vi "CameraSetParams.vi"(8 "error in (no error)":errorcluster, 10 "settings":T2={"exposure"=0.0, "external"=FALSE, "roi"={"left"=0, "top"=0, "right"=0, "bottom"=0}, "frames"=0, "bin_x"=1, "bin_y"=1}, 11 "NIvision in":refnum<class "IMAQdx.lvclass">) -> (0 "error out":errorcluster, 1 "roi_out":T1, 2 "attributes":variant[](array[variant]), 3 "NIvision out":refnum<class "IMAQdx.lvclass">)   [LabVIEW 2010, in "IMAQdx.lvclass"]
uses:
  IMAQdx.lvclass
  subvis/ExposureSettings.ctl
  subvis/ROI_rect.ctl
  <vilib>/vision/driver/IMAQdx.llb/IMAQdx Acquisition Mode.ctl
  IMAQdx.lvclass/IMAQdx.ctl
  <vilib>/vision/driver/NI_Vision_Acquisition_Software.lvlib
  Program Files (x86)/National Instruments/LabVIEW 2010/resource/objmgr/imaqdx.rc
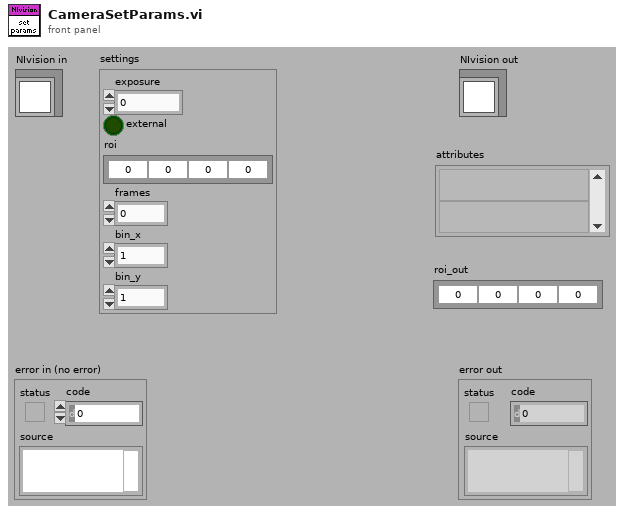
[diagram p1: front panel]
types:
  T1 = typedef "ROI_rect.ctl" = cluster{"left":i32, "top":i32, "right":i32, "bottom":i32}
  T2 = typedef "ExposureSettings.ctl" = cluster{"exposure":dbl, "external":bool, "roi":T1, "frames":i32, "bin_x":u8, "bin_y":u8}
  T3 = typedef "NI_Vision_Acquisition_Software.lvlib/IMAQdx Acquisition Mode.ctl" = enum32{"One Shot", "Continuous"}
  T4 = typedef "IMAQdx.ctl" = refnum<k21>
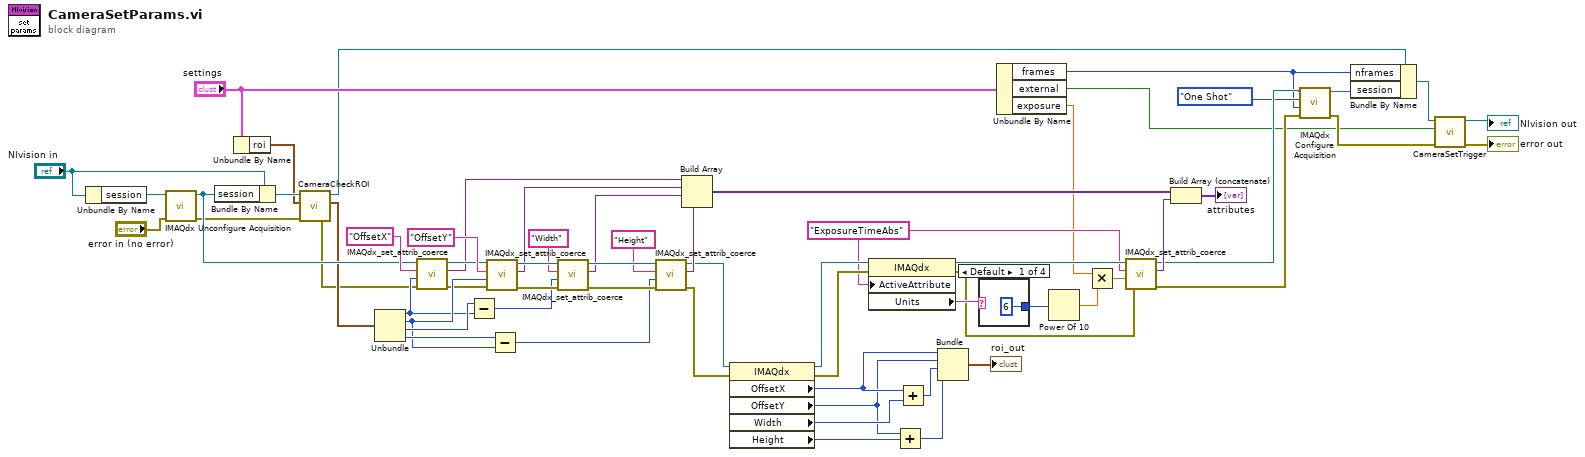
[diagram p0: block diagram]
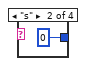
[diagram p2: hidden frame]
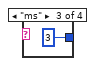
[diagram p3: hidden frame]
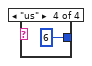
[diagram p4: hidden frame]
diagram:
  w27 = "ExposureTimeAbs" ("ActiveAttribute")
  n1 = Unbundle By Name("NIvision in") -> ("session"=w24:refnum<k21>)
  n2 = call <vilib>:"IMAQdx Unconfigure Acquisition.vi"("error in"="error in (no error)", "Session In"=w24) -> ("error out"=w7:errorcluster, "Session Out"=w13:T4)  [unwired: 8 in]
  n3 = Bundle By Name(cluster="NIvision in", "session"=w13) -> (w11:refnum<class "IMAQdx.lvclass">)
  n4 = Unbundle By Name("settings") -> ("roi"=w9:T1)
  n5 = call-dynamic "CameraCheckROI.vi"("error in (no error)"=w7, "ROI_in"=w9, "IMAQdx in"=w11) -> ("error out"=w6:errorcluster, "ROI_out"=w8:T1, "IMAQdx out"=w10:refnum<class "IMAQdx.lvclass">)  [unwired: 6 in]
  n6 = Unbundle(w8) -> ("left"=w53:i32, "top"=w57:i32, "right"=w63:i32, "bottom"=w60:i32)
  n7 = call "IMAQdx_set_attrib_coerce.vi"("error in"=w6, "value"=w53, "attribute"="OffsetX", "IMAQdx in"=w13) -> ("error out"=w56:errorcluster, "attrib out"=w54:variant, "IMAQdx out"=w55:T4)  [unwired: 1 out]
  n8 = Subtract(x=w63, y=w53) -> (x-y=w48:i32)
  n9 = call "IMAQdx_set_attrib_coerce.vi"("error in"=w56, "value"=w57, "attribute"="OffsetY", "IMAQdx in"=w55) -> ("error out"=w51:errorcluster, "attrib out"=w46:variant, "IMAQdx out"=w52:T4)  [unwired: 1 out]
  n10 = Subtract(x=w60, y=w57) -> (x-y=w47:i32)
  n11 = call "IMAQdx_set_attrib_coerce.vi"("error in"=w51, "value"=w48, "attribute"="Width", "IMAQdx in"=w52) -> ("error out"=w49:errorcluster, "attrib out"=w45:variant, "IMAQdx out"=w50:T4)  [unwired: 1 out]
  n12 = call "IMAQdx_set_attrib_coerce.vi"("error in"=w49, "value"=w47, "attribute"="Height", "IMAQdx in"=w50) -> ("error out"=w32:errorcluster, "attrib out"=w44:variant, "IMAQdx out"=w30:T4)  [unwired: 1 out]
  n13 = Build Array(w54, w46, w45, w44) -> (w41:variant[])
  n14 = property class="IMAQdx"(reference=w30, error in=w32) -> (reference out=w29:T4, error out=w31:errorcluster, "OffsetX"=w38:u32, "OffsetY"=w37:u32, "Width"=w39:u32, "Height"=w40:u32)
  n15 = property class="IMAQdx"(reference=w29, error in=w31, "ActiveAttribute"=w27) -> (reference out=w28:T4, error out=w26:errorcluster, "Units"=w61:string)
  n16 = Add(x=w37, y=w40) -> (x+y=w35:u32)
  n17 = Add(x=w38, y=w39) -> (x+y=w36:u32)
  n18 = Bundle("OffsetX"=w38, "OffsetY"=w37, w36, w35) -> (→"roi_out":cluster{"OffsetX":u32, "OffsetY":u32, u32, u32})  [unwired: 1 in]
  n19 = case shown="Default" w61 {
    tunnel: [6 ("y") 0 ("y") 3 ("y") 6 ("y")] -> w4
    frame Default {
    }
    frame "s" {
    }
    frame "ms" {
    }
    frame "us" {
    }
  }
  n20 = Unbundle By Name("settings") -> ("frames"=w15:i32, "external"=w12:bool, "exposure"=w1:dbl)
  n21 = Power Of 10(x=w4) -> (10^x=w3:dbl)
  n22 = Multiply(x=w1, y=w3) -> (x*y=w2:dbl)
  n23 = call "IMAQdx_set_attrib_coerce.vi"("error in"=w26, "value"=w2, "attribute"=w27, "IMAQdx in"=w28) -> ("error out"=w17:errorcluster, "attrib out"=w25:variant, "IMAQdx out"=w19:T4)  [unwired: 1 out]
  n24 = Build Array (concatenate)(w41, w25) -> (→"attributes":variant[])
  n25 = call <vilib>:"IMAQdx Configure Acquisition.vi"("error in"=w17, "Number of Buffers"=w15, "Continuous?"=IMAQdx_Acquisition_Mode."One Shot", "Session In"=w19) -> ("error out"=w16:errorcluster, "Session Out"=w20:T4)  [unwired: 6 in]
  n26 = Bundle By Name(cluster=w10, "nframes"=w15, "session"=w20) -> (w5:refnum<class "IMAQdx.lvclass">)
  n27 = call-dynamic "CameraSetTrigger.vi"("error in (no error)"=w16, "external?"=w12, "IMAQdx in"=w5) -> ("error out"=→"error out":errorcluster, "IMAQdx out"=→"NIvision out":refnum<class "IMAQdx.lvclass">)  [unwired: 6 in, 1 out]
